vi "Value.vi"(8 "error in (no error)":errorcluster, 11 "Channel BOOL in":refnum<class "Channel BOOL.lvclass">) -> (0 "error out":errorcluster, 1 "Timestamp":dbl, 2 "Scaled":bool, 3 "Channel BOOL out":refnum<class "Channel BOOL.lvclass">, 4 "Raw":bool)   [LabVIEW 2020, in "Vecto.lvlib" / "Channel BOOL.lvclass"]
uses:
  Channel BOOL.lvclass
  Channel BOOL.lvclass/Channel BOOL.ctl
  Group BOOL/Group BOOL.lvclass
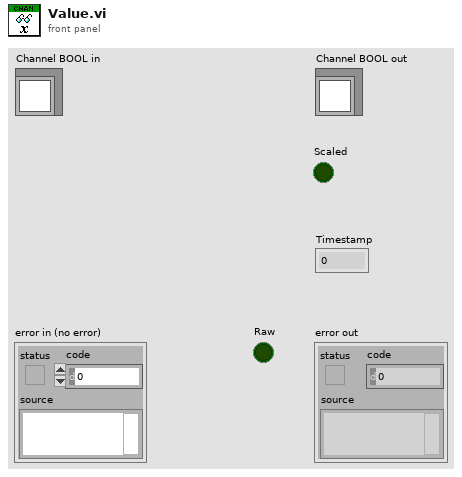
[diagram p1: front panel]
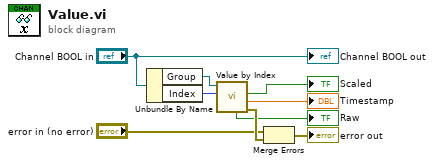
[diagram p0: block diagram]
diagram:
  n1 = Unbundle By Name("Channel BOOL in") -> ("Group"=w9:refnum<class "Group BOOL.lvclass">, "Index"=w8:i32)
  n2 = call "Value by Index.vi"("Index"=w8, "Group BOOL in"=w9) -> ("error out"=w7:errorcluster, "Timestamp"=→"Timestamp":dbl, "Scaled"=→"Scaled":bool, "Raw"=→"Raw":bool)  [unwired: 5 in, 1 out]
  n3 = Merge Errors("error in (no error)", w7) -> (→"error out":errorcluster)
  "Channel BOOL out" <- "Channel BOOL in"
